vi "DATA_RSHP.vi"(1 "Digital in":refnum<vi>, 2 "data in":string) -> (0 "DATA FRAME":string)   [LabVIEW 2013]
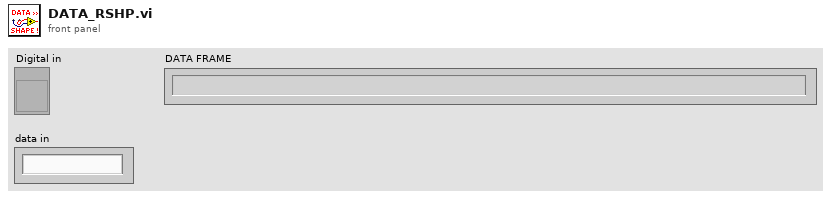
[diagram p1: front panel]
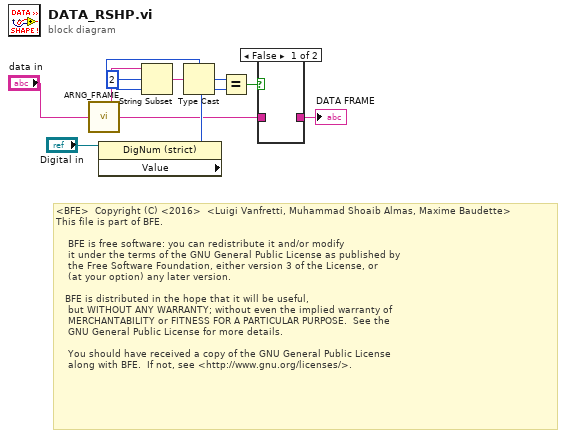
[diagram p0: block diagram]
diagram:
  w5 = u16 2 ("offset (0)")
  # "<BFE>  Copyright (C) <2016>  <Luigi Vanfretti, Muhammad Shoaib Almas, Maxime Baudette> \nThis file is part of BFE.\n\n    BFE is free software: you can redistribute it and/or modify\n    it under the terms of the GNU General Public License as published by\n    the Free Software Foundation, either version 3 of the License, or\n    (at your option) any later version.\n\n   BFE is distributed in the hope that it will be useful,\n    but WITHOUT ANY WARRANTY; without even the implied warranty of\n    MERCHANTABILITY or FITNESS FOR A PARTICULAR PURPOSE.  See the\n    GNU General Public License for more details.\n\n    You should have received a copy of the GNU General Public License\n    along with BFE.  If not, see <http://www.gnu.org/licenses/>."
  n1 = call "ARNG_FRAME.vi"("DATA FRAME"="data in") -> ("Arranged Data"=w4:string)
  n2 = property class="DigNum (strict)"(reference="Digital in") -> ("Value"=w8:u32)  [unwired: 1 in, 2 out]
  n3 = String Subset(string=w4, offset (0)=w5, length (rest)=w5) -> (substring=w6:string)
  n4 = Type Cast(type=w5, x=w6) -> (*(type *) &x=w7:u16)
  n5 = Equal?(x=w7, y=w8) -> (x = y?=w9:bool)
  n6 = case shown="False" w9 {
    tunnel: [_ w10] -> w3
    tunnel: w4 -> [_ w10]
    frame False {
    }
    frame True {
    }
  }
  "DATA FRAME" <- w3
